vi "Read Input.vi"(11 "Path":path=path "D:/gitRepo/AdventofCode-2020-LabVIEW/Inputs/Day 4.txt") -> (3 "string array":string[](array[string]))   [LabVIEW 2020]
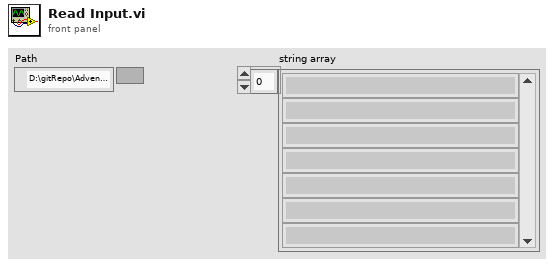
[diagram p1: front panel]
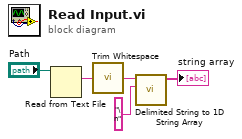
[diagram p0: block diagram]
diagram:
  n1 = Read from Text File(file (use dialog)="Path") -> (text=w3:string)  [unwired: 3 in, 3 out]
  n2 = call <vilib>:"Trim Whitespace.vi"("string"=w3) -> ("trimmed string"=w2:string)  [unwired: 1 in]
  n3 = call <vilib>:"Delimited String to 1D String Array.vi"("delimiter"="\n", "delimited string"=w2) -> ("string array"=→"string array":string[])  [unwired: 9 in]
